vi "Xeryon send serial data.vi"(4 "Data to send":string) -> ()   [LabVIEW 2019]
uses:
  Xeryon serial command.ctl
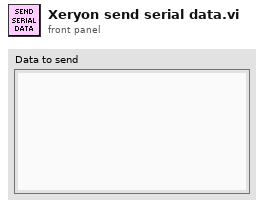
[diagram p1: front panel]
types:
  T1 = typedef "Xeryon serial command.ctl" = cluster{"Command":enum16{"Send serial data", "Exit"}, "Data to send":string}
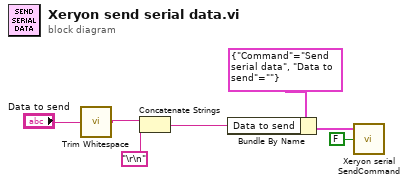
[diagram p0: block diagram]
diagram:
  n1 = call <vilib>:"Trim Whitespace.vi"("string"="Data to send") -> ("trimmed string"=w3:string)  [unwired: 1 in]
  n2 = Concatenate Strings(w3, "\r\n") -> (w1:string)
  n3 = Bundle By Name(cluster=T1 {"Command"=enum."Send serial data", "Data to send"=""} ("Serial Message"), "Data to send"=w1) -> (w6:T1)
  n4 = call "Xeryon serial SendCommand.vi"("Feedback?"=FALSE, "Serial Command"=w6) -> ()  [unwired: 1 in, 3 out]
